vi "Abort.vi"(11 "messengerMbase in":refnum<class "MessengerMBase.lvclass">) -> (3 "messengerMbase out":refnum<class "MessengerMBase.lvclass">)   [LabVIEW 2019, in "MessengerM.lvlib" / "MessengerMBase.lvclass"]
uses:
  MessengerMBase.lvclass
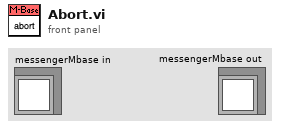
[diagram p1: front panel]
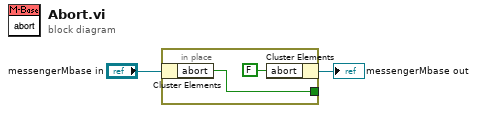
[diagram p0: block diagram]
diagram:
  n1 = in-place {
    in-place-border: [w3] -> _
    n2 = in-place-cluster #1("messengerMbase in") -> ("abort"=w3:bool)
    n3 = in-place-cluster #1("abort"=FALSE) -> (→"messengerMbase out":refnum<class "MessengerMBase.lvclass">)
  }
